vi "Get Popup.vi"(8 "error in (no error)":errorcluster caption="错误输入（无错误）", 10 "Point":T1, 11 "Popup 输入":refnum<class "Popup.lvclass"> caption="DNL_LabVIEW Object in") -> (0 "error out":errorcluster caption="错误输出", 3 "Popup 输出":refnum<class "Popup.lvclass"> caption="DNL_LabVIEW Object out")   [LabVIEW 2017, in "Popup.lvclass"]
uses:
  Popup.lvclass
  <vilib>/Utility/miscctls.llb/LVPositionTypeDef.ctl
  Popup.lvclass/Popup.ctl
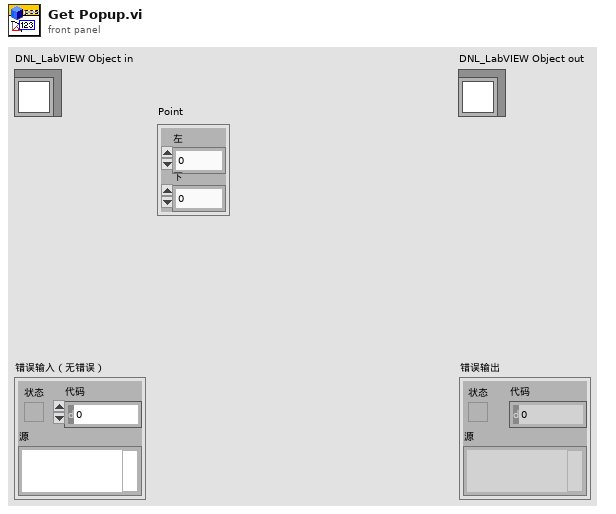
[diagram p1: front panel]
types:
  T1 = typedef "LVPositionTypeDef.ctl" = cluster{"Left":i32, "Top":i32}
  T2 = typedef "LVRowAndColumnTypeDef.ctl" = cluster{"Row":i32, "Column":i32}
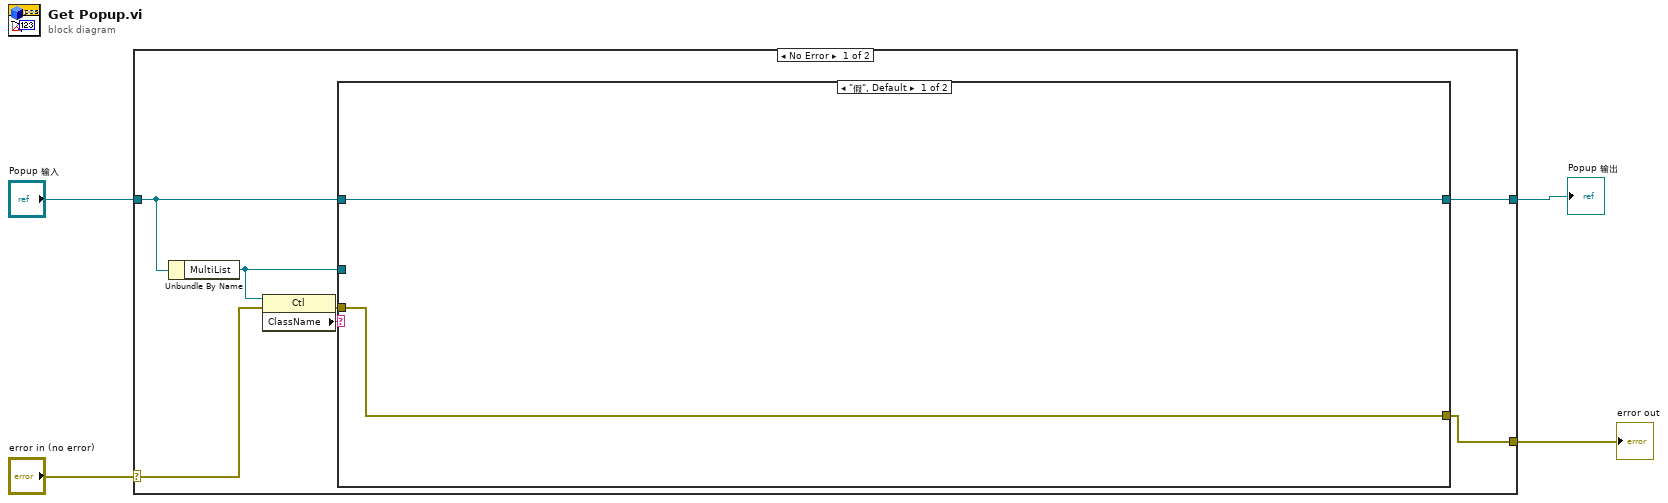
[diagram p0: block diagram]
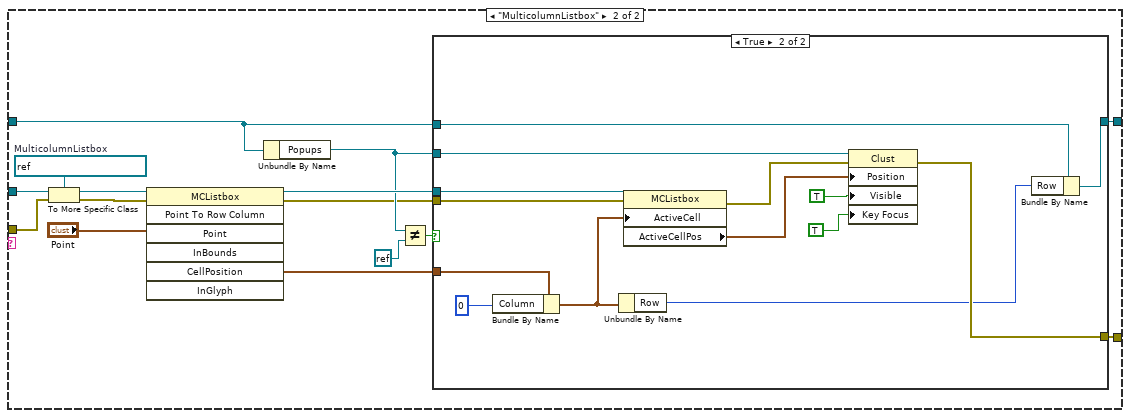
[diagram p2: hidden frame]
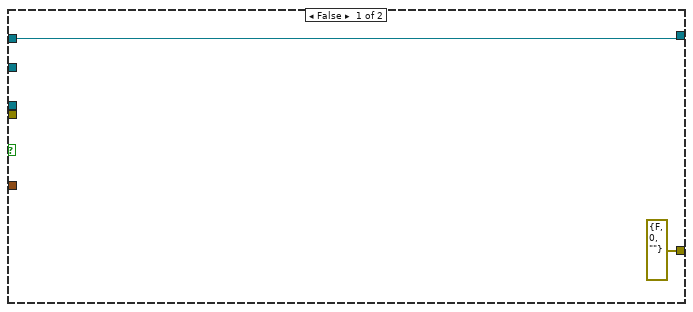
[diagram p3: hidden frame]
diagram:
  n1 = case shown="No Error" "error in (no error)" {
    selector: "error in (no error)" -> [w8 w46]
    tunnel: [w5 w46] -> w3
    tunnel: [w10 w45] -> w1
    tunnel: "Popup 输入" -> [w11 w45]
    frame No Error {
      n2 = Unbundle By Name(w11) -> ("MultiList"=w9:refnum<vi>)
      n3 = property class="Ctl"(reference=w9, error in=w8) -> (error out=w6:errorcluster, "ClassName"=w7:string)  [unwired: 1 out]
      n4 = case shown="\"假\", Default" w7 {
        tunnel: w11 -> [w13 w24]
        tunnel: [w12 w22] -> w5
        tunnel: [w13 w21] -> w10
        tunnel: w9 -> [_ w20]
        tunnel: w6 -> [w12 w19]
        frame "假", Default {
        }
        frame "MulticolumnListbox" {
          w28 = refnum<vi> refnum  # MulticolumnListbox
          n5 = To More Specific Class(target class=w28, reference=w20, error in=w19) -> (specific class reference=w27:refnum<vi>, error out=w26:errorcluster)
          n6 = invoke class="MCListbox" method="Point To Row Column"(reference=w27, error in=w26, "Point"="Point") -> (reference out=w23:refnum<vi>, error out=w15:errorcluster, "CellPosition"=w14:T2)  [unwired: 4 in, 4 out]
          n7 = Unbundle By Name(w24) -> ("Popups"=w16:refnum<vi>)
          n8 = Not Equal?(x=w16, y=refnum<k0> refnum) -> (x != y?=w18:bool)
          n9 = case shown="True" w18 {
            tunnel: w24 -> [w30 w42]
            tunnel: w23 -> [_ w44]
            tunnel: [errorcluster {"status"=FALSE, "code"=0, "source"=""} ("error out") w43] -> w22
            tunnel: [w30 w41] -> w21
            tunnel: w14 -> [_ w34]
            tunnel: w16 -> [_ w37]
            tunnel: w15 -> [_ w36]
            frame False {
            }
            frame True {
              n10 = Bundle By Name(cluster=w34, "Column"=0) -> (w32:T2)
              n11 = Unbundle By Name(w32) -> ("Row"=w31:i32)
              n12 = property class="MCListbox"(reference=w44, error in=w36, "ActiveCell"=w32) -> (error out=w40:errorcluster, "ActiveCellPos"=w35:T1)  [unwired: 1 out]
              n13 = property class="Clust"(reference=w37, error in=w40, "Position"=w35, "Visible"=TRUE, "Key Focus"=TRUE) -> (error out=w43:errorcluster)  [unwired: 1 out]
              n14 = Bundle By Name(cluster=w42, "Row"=w31) -> (w41:refnum<class "Popup.lvclass">)
            }
          }
        }
      }
    }
    frame Error {
    }
  }
  "error out" <- w3
  "Popup 输出" <- w1
